vi "Steering Type String to Enum.vi"(11 "steering type_string":string) -> (2 "found?":bool, 3 "steering type_enum":T1 items=["User Defined", "Differential", "Ackermann", "Mecanum"])   [LabVIEW 2017, in "NI_Robotics_Configure Steering Frame.lvlib"]
uses:
  <vilib>/robotics/Dialog/Configure Steering Frame/NI_Robotics_Configure Steering Frame.lvlib
  <vilib>/robotics/Dialog/Configure Steering Frame/Steering Type.ctl
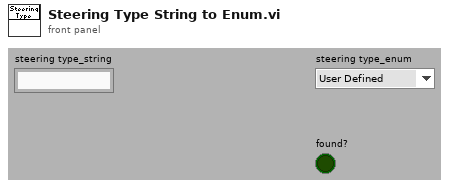
[diagram p1: front panel]
types:
  T1 = typedef "NI_Robotics_Configure Steering Frame.lvlib/Steering Type.ctl" = u16
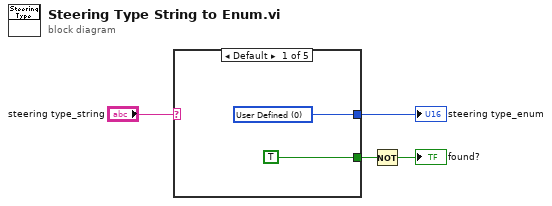
[diagram p0: block diagram]
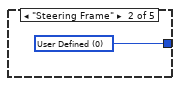
[diagram p2: hidden frame]
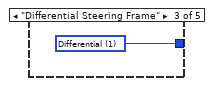
[diagram p3: hidden frame]
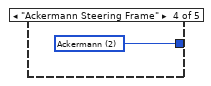
[diagram p4: hidden frame]
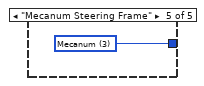
[diagram p5: hidden frame]
diagram:
  n1 = case shown="Default" "steering type_string" {
    tunnel: [w6 w7 w8 w9 w10] -> w3
    tunnel: [TRUE _ _ _ _] -> w2
    frame Default {
      w6 = T1 0 items=["User Defined", "Differential", "Ackermann", "Mecanum"] ("steering type_enum")
    }
    frame "Steering Frame" {
      w7 = T1 0 items=["User Defined", "Differential", "Ackermann", "Mecanum"] ("steering type_enum")
    }
    frame "Differential Steering Frame" {
      w8 = T1 1 items=["User Defined", "Differential", "Ackermann", "Mecanum"] ("steering type_enum")
    }
    frame "Ackermann Steering Frame" {
      w9 = T1 2 items=["User Defined", "Differential", "Ackermann", "Mecanum"] ("steering type_enum")
    }
    frame "Mecanum Steering Frame" {
      w10 = T1 3 items=["User Defined", "Differential", "Ackermann", "Mecanum"] ("steering type_enum")
    }
  }
  "steering type_enum" <- w3
  n2 = Not(x=w2) -> (.not. x?=→"found?":bool)
